vi "Modulation.vi"(0 "Parameters":T1={"Deadtime"="Deadtime", "Period"="Period", "A_timing"="A_timing", "B_timing"="B_timing", "C_timing"="C_timing"}, 11 "enable":bool=TRUE) -> (4 "SwitchPositions":T2)   [LabVIEW 2017, in "SVPWM.lvlib"]
uses:
  SVPWM.lvlib
  SwitchPositions.ctl
  Parameters.ctl
  <vilib>/Utility/error.llb/Clear Errors.vi
  <vilib>/rvi/Emulation/niFpgaSctlEmulationGetInTimedLoop.vi
  <vilib>/rvi/DataTransferAndStorage/Container/Common/niFpgaContainerExecOnDevCompGetState.vi
  <vilib>/rvi/Emulation/niFpgaEmulationIsFPGAContextNoSignature.vi
  <vilib>/rvi/DataTransferAndStorage/Container/Common/niFpgaContainerGetUniqueNameForEmu.vi
  <vilib>/rvi/Memory/Memory_Emulation/niFpgaMemoryEmulationCacheClearOnFirstRun.vi
  <vilib>/rvi/Memory/Memory_Emulation/nirvimemoryEmulationManagerCache_MakeExclusive.vi
  <vilib>/rvi/Memory/Memory_Emulation/niFpgaMemoryEmulationValidateCache.vi
  <vilib>/rvi/Memory/Memory_Emulation/nirvimemoryEmulationManagerCache_InsertValue.vi
  <vilib>/rvi/Memory/Memory_Emulation/nirvimemoryEmulationManagerCache_ReleaseExclusive.vi
  <vilib>/rvi/Memory/Memory_Emulation/nirvimemoryEmulationManagerCache_GetValue.vi
  <vilib>/rvi/Memory/Memory_Emulation/nirvimemoryEmulationManagerCache_SetValue.vi
  <vilib>/rvi/Emulation/niFpgaProcessEmulError.vi
  <vilib>/rvi/DataTransferAndStorage/Container/XNode/niFpgaContainer.xnode
  <vilib>/rvi/DataTransferAndStorage/Register/Emulation/niFpgaRegisterEmulationRefIn.vi
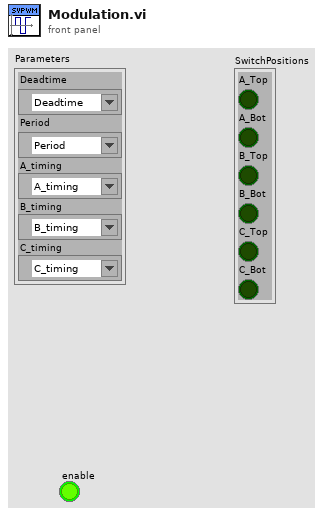
[diagram p1: front panel]
types:
  T1 = typedef "SVPWM.lvlib/Parameters.ctl" = cluster{"Deadtime":refnum<k21>, "Period":refnum<k21>, "A_timing":refnum<k21>, "B_timing":refnum<k21>, "C_timing":refnum<k21>}
  T2 = typedef "SVPWM.lvlib/SwitchPositions.ctl" = cluster{"A_Top":bool, "A_Bot":bool, "B_Top":bool, "B_Bot":bool, "C_Top":bool, "C_Bot":bool}
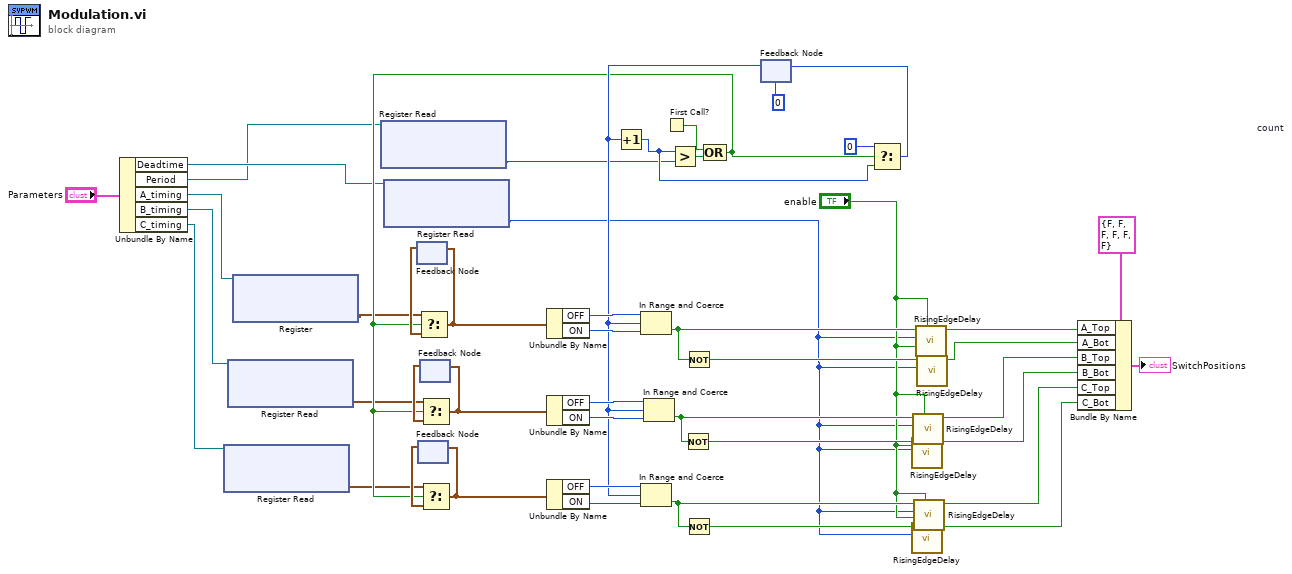
[diagram p0: block diagram]
diagram:
  n1 = Unbundle By Name("Parameters") -> ("Deadtime"=w4:refnum<k21>, "Period"=w2:refnum<k21>, "A_timing"=w10:refnum<k21>, "B_timing"=w8:refnum<k21>, "C_timing"=w6:refnum<k21>)
  n2 = xnode "Register Read"("Register In"=w6) -> ("Data"=w5:cluster{"ON":u32, "OFF":u32})  [unwired: 1 out]
  n3 = xnode "Register Read"("Register In"=w8) -> ("Data"=w7:cluster{"ON":u32, "OFF":u32})  [unwired: 1 out]
  n4 = xnode "Register"("Register In"=w10) -> ("Data"=w9:cluster{"ON":u32, "OFF":u32})  [unwired: 1 out]
  n5 = xnode "Register Read"("Register In"=w2) -> ("Data"=w1:u32)  [unwired: 1 out]
  n6 = xnode "Register Read"("Register In"=w4) -> ("Data"=w3:u8)  [unwired: 1 out]
  n7 = feedback #1() -> (w20:cluster{"ON":u32, "OFF":u32})  [unwired: 1 in]
  n8 = feedback #2() -> (w17:cluster{"ON":u32, "OFF":u32})  [unwired: 1 in]
  n9 = feedback #3() -> (w19:cluster{"ON":u32, "OFF":u32})  [unwired: 1 in]
  n10 = First Call?() -> (First Call?: T/F=w12:bool)
  n11 = feedback #4 "count"(u32 0 ("Period")) -> (w32:u32)
  n12 = Increment(x=w32) -> (x+1=w45:u32)
  n13 = Greater?(x=w45, y=w1) -> (0:w14:bool)
  n14 = Compound Arithmetic op=OR(w12, w14) -> (w13:bool)
  n15 = Select(t=w9, s=w13, f=w20) -> (s? t:f=w15:cluster{"ON":u32, "OFF":u32})
  n16 = feedback-in #1(w15) -> ()
  n17 = Select(t=w7, s=w13, f=w19) -> (s? t:f=w18:cluster{"ON":u32, "OFF":u32})
  n18 = feedback-in #3(w18) -> ()
  n19 = Select(t=w5, s=w13, f=w17) -> (s? t:f=w16:cluster{"ON":u32, "OFF":u32})
  n20 = feedback-in #2(w16) -> ()
  n21 = Unbundle By Name(w15) -> ("OFF"=w42:u32, "ON"=w41:u32)
  n22 = Unbundle By Name(w18) -> ("OFF"=w37:u32, "ON"=w38:u32)
  n23 = Unbundle By Name(w16) -> ("OFF"=w34:u32, "ON"=w33:u32)
  n24 = In Range and Coerce(upper limit=w42, x=w32, lower limit=w41) -> (In Range?=w39:bool)  [unwired: 1 out]
  n25 = In Range and Coerce(upper limit=w34, x=w32, lower limit=w33) -> (In Range?=w31:bool)  [unwired: 1 out]
  n26 = In Range and Coerce(upper limit=w37, x=w32, lower limit=w38) -> (In Range?=w35:bool)  [unwired: 1 out]
  n27 = Not(x=w35) -> (.not. x?=w36:bool)
  n28 = Not(x=w39) -> (.not. x?=w40:bool)
  n29 = Not(x=w31) -> (.not. x?=w30:bool)
  n30 = Select(t=u32 0, s=w13, f=w45) -> (s? t:f=w43:u32)
  n31 = feedback-in #4(w43) -> ()
  n32 = call "RisingEdgeDelay.vi"("enable?"="enable", "Deadtime (iterations)"=w3, "Input"=w36) -> ("Output"=w24:bool)  [unwired: 8 in]
  n33 = call "RisingEdgeDelay.vi"("enable?"="enable", "Deadtime (iterations)"=w3, "Input"=w30) -> ("Output"=w22:bool)  [unwired: 8 in]
  n34 = call "RisingEdgeDelay.vi"("enable?"="enable", "Deadtime (iterations)"=w3, "Input"=w35) -> ("Output"=w25:bool)  [unwired: 8 in]
  n35 = call "RisingEdgeDelay.vi"("enable?"="enable", "Deadtime (iterations)"=w3, "Input"=w31) -> ("Output"=w23:bool)  [unwired: 8 in]
  n36 = call "RisingEdgeDelay.vi"("enable?"="enable", "Deadtime (iterations)"=w3, "Input"=w39) -> ("Output"=w27:bool)  [unwired: 8 in]
  n37 = call "RisingEdgeDelay.vi"("enable?"="enable", "Deadtime (iterations)"=w3, "Input"=w40) -> ("Output"=w26:bool)  [unwired: 8 in]
  n38 = Bundle By Name(cluster=T2 {"A_Top"=FALSE, "A_Bot"=FALSE, "B_Top"=FALSE, "B_Bot"=FALSE, "C_Top"=FALSE, "C_Bot"=FALSE} ("SwitchPositions"), "A_Top"=w27, "A_Bot"=w26, "B_Top"=w25, "B_Bot"=w24, "C_Top"=w23, "C_Bot"=w22) -> (→"SwitchPositions":T2)
